vi "PSCHN_Update Variable.vi"(6 "data":cluster{"Tag":string, "Popup Value":variant}, 8 "error in (no error)":errorcluster, 9 "PopUp Para":T5, 10 "Cards":T1[](array[typedef]), 11 "Tree":refnum<vi>) -> (0 "error out":errorcluster, 2 "Cards Out":T1[](array[typedef]))   [LabVIEW 2016]
uses:
  Controls/PSCHN_Card Para.ctl
  Controls/PSCHN_Channel Para.ctl
  <vilib>/Pansino Software/ToolkitLib/Popup Toolkit/Private/Ctrls/PSPOP_Grid.Cell Info.ctl
  <vilib>/Pansino Software/ToolkitLib/Popup Toolkit/Private/Ctrls/PSPOP_Data Type.ctl
panel:
  in  "Cell Info (type only)":T3={"Tag"="", "Row"=0, "Column"=0, "In Symbol?"=FALSE, "In Data?"=FALSE, "Cell String"="", "Ctl Refnum"=refnum, "Prop Type"=enum."Unkown", "Ring Strings"=[], "Ring Values"=[], "New Cell String"=""}
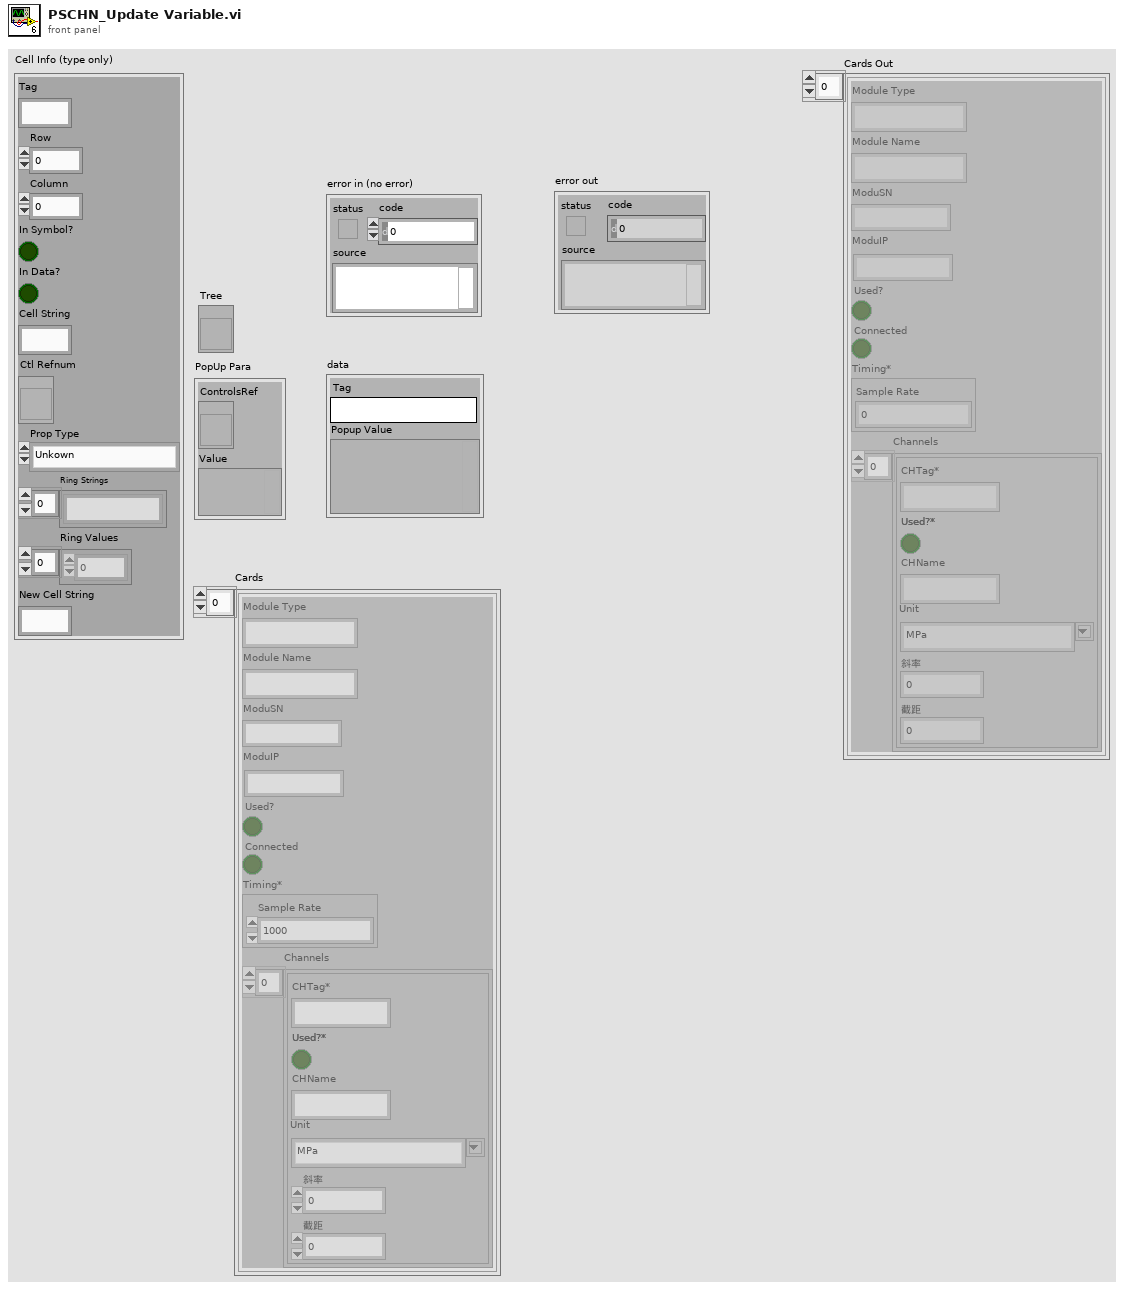
[diagram p1: front panel]
types:
  T1 = typedef "PSCHN_Card Para.ctl" = cluster{"Module Type":string, "Module Name":string, "ModuSN":string, "ModuIP":string, "Used?":bool, "Connected":bool, "Timing*":cluster{"Sample Rate":dbl}, "Channels":T2[]}
  T2 = typedef "PSCHN_Channel Para.ctl" = cluster{"CHTag*":string, "Used?*":bool, "CHName":string, "Unit":string, "斜率":dbl, "截距":dbl}
  T3 = typedef "PSPOP_Grid.Cell Info.ctl" = cluster{"Tag":string, "Row":i32, "Column":i32, "In Symbol?":bool, "In Data?":bool, "Cell String":string, "Ctl Refnum":refnum<vi>, "Prop Type":T4, "Ring Strings":string[], "Ring Values":ext[], "New Cell String":string}
  T4 = typedef "PSPOP_Data Type.ctl" = enum16{"NO POPUP", "Unkown", "String", "Integer", "Float", "Color", "Boolean", "Ring", "Captioned String", "Captioned Integer", "Button Color", "2 Int Cluster", "4 Int Cluster", "6-Dbl Cluster", "Path", "Combox", "Time", "ShotCut String"}
  T5 = cluster{"ControlsRef":refnum<vi>, "Value":variant}
  T6 = typedef "PSCFO_ParaDataType.ctl" = cluster{"ParaTag":string, "ParaName":string, "ParaType":string, "PicName":string, "ParaLevel":string, "DefaultValue":variant, "ParaVisable?":bool, "ParaOperation?":bool, "Operation":cluster{"ParaValue":string, "Operation":cluster{"ChangePara":cluster{"ParaName":string, "ParaData":string}[], "EnablePara":string[]}}[], "Ring Para":T7}
  T7 = typedef "PSLIST_Para Related.ctl" = cluster{"Strings":string[], "Values":ext[], "Use":bool, "Combox":string[], "Browse Options":T8, "Combo Box":cluster{"Allow Undefined Strings":bool}}
  T8 = typedef "LVBrowseOptionsTypeDef.ctl" = cluster{"Prompt":string, "Match Pattern":string, "Mode":enum32{"existing file", "new file", "new or existing file", "existing dir", "new dir", "new or existing dir", "existing file (use LLBs)", "new file (use LLBs)", "new or existing file (use LLBs)", "new or existing file or directory (use LLBs)", "existing dir (use LLBs)", "new dir (use LLBs)", "new or existing dir (use LLBs)", "existing file or dir", "new file or dir", "new or existing file or dir", "existing file or dir (use LLBs)", "new file or dir (use LLBs)"}, "Start Path":path, "Pattern Label":string, "Button Text":string}
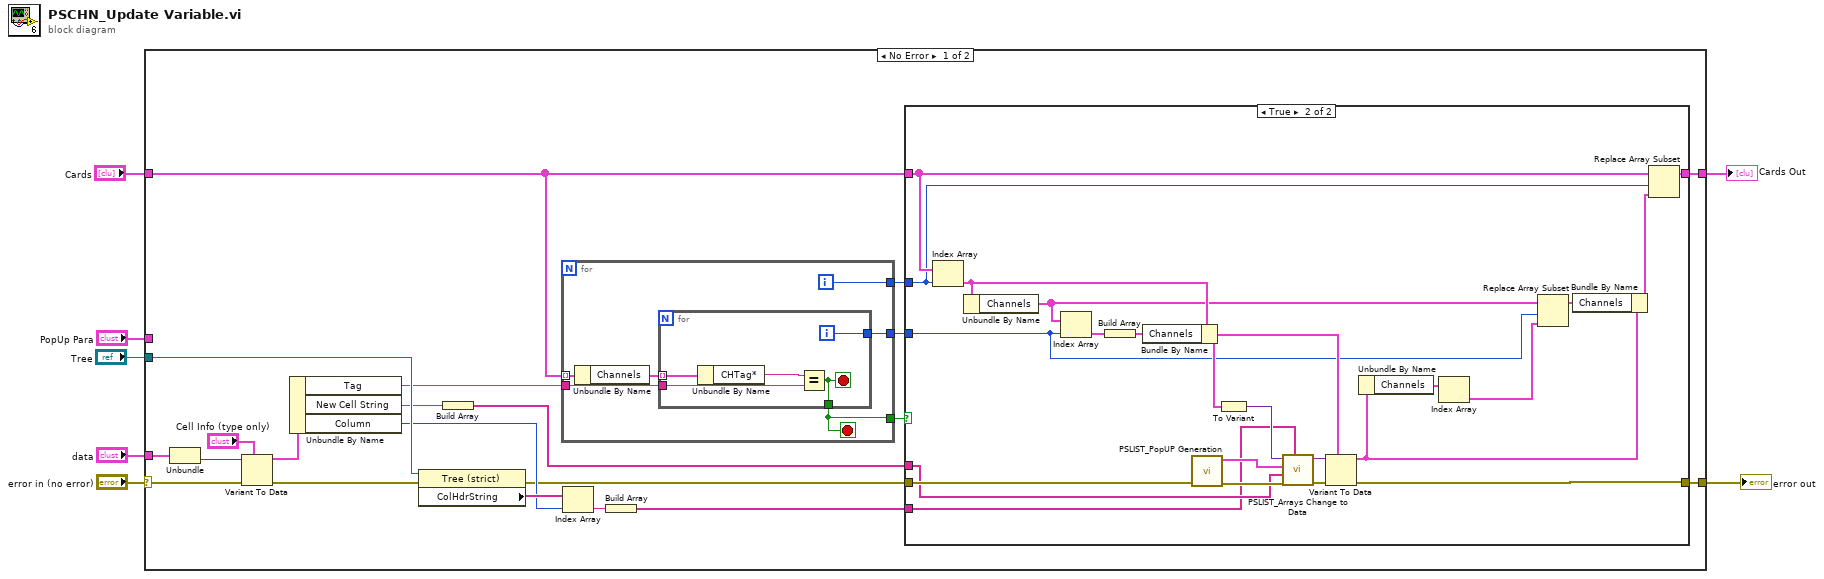
[diagram p0: block diagram]
diagram:
  n1 = case shown="No Error" "error in (no error)" {
    selector: "error in (no error)" -> [w27 w66]
    tunnel: [w12 w66] -> w7
    tunnel: "PopUp Para" -> [_ _]
    tunnel: "Cards" -> [w15 w65]
    tunnel: "data" -> [w28 _]
    tunnel: "Tree" -> [w23 _]
    tunnel: [w14 w65] -> w1
    frame No Error {
      n2 = Unbundle(w28) -> ("Popup Value"=w26:variant)  [unwired: 1 out]
      n3 = Variant To Data(error in=w27, type="Cell Info (type only)", Variant=w26) -> (data=w24:T3, error out=w22:errorcluster)
      n4 = Unbundle By Name(w24) -> ("Tag"=w19:string, "New Cell String"=w18:string, "Column"=w20:i32)
      n5 = property class="Tree (strict)"(reference=w23, error in=w22) -> (error out=w13:errorcluster, "ColHdrString"=w21:string[])  [unwired: 1 out]
      n6 = Build Array(w18) -> (w8:string[])
      n7 = for {
        tunnel: w15 -> [w57] mode=indexing
        tunnel: w19 -> [w58]
        tunnel: [w56] -> w10
        tunnel: [w55] -> w11
        tunnel: [w54] -> w16
        i -> [w55]
        stop <- w54 stop-if-true
        n8 = Unbundle By Name(w57) -> ("Channels"=w59:T2[])
        n9 = for {
          tunnel: w59 -> [w62] mode=indexing
          tunnel: w58 -> [w63]
          tunnel: [w61] -> w54
          tunnel: [w60] -> w56
          i -> [w60]
          stop <- w61 stop-if-true
          n10 = Unbundle By Name(w62) -> ("CHTag*"=w64:string)
          n11 = Equal?(x=w64, y=w63) -> (x = y?=w61:bool)
        }
      }
      n12 = Index Array(array=w21, index=w20) -> (element=w17:string)
      n13 = Build Array(w17) -> (w9:string[])
      n14 = case shown="True" w16 {
        tunnel: w15 -> [w30 w37]
        tunnel: [w30 w34] -> w14
        tunnel: w13 -> [w29 w50]
        tunnel: [w29 w32] -> w12
        tunnel: w11 -> [_ w36]
        tunnel: w10 -> [_ w40]
        tunnel: w9 -> [_ w33]
        tunnel: w8 -> [_ w42]
        frame False {
        }
        frame True {
          n15 = Index Array(array=w37, index=w36) -> (element=w51:T1)
          n16 = Unbundle By Name(w51) -> ("Channels"=w41:T2[])
          n17 = Index Array(array=w41, index=w40) -> (element=w52:T2)
          n18 = Build Array(w52) -> (w53:T2[])
          n19 = Bundle By Name(cluster=w51, "Channels"=w53) -> (w49:T1)
          n20 = call <vilib>:"PSLIST_PopUP Generation.vi"("错误输入（无错误）"=w50) -> ("error out"=w45:errorcluster, "PopUpPara"=w44:T6[])  [unwired: 9 in]
          n21 = To Variant(anything=w49) -> (Variant=w46:variant)
          n22 = call <vilib>:"PSLIST_Arrays Change to Data.vi"("Column Headers"=w33, "Error In"=w45, "Column Strings"=w42, "Parameter"=w44, "VData"=w46) -> ("Error Out"=w47:errorcluster, "Data Out"=w48:variant)  [unwired: 4 in, 1 out]
          n23 = Variant To Data(error in=w47, type=w49, Variant=w48) -> (data=w39:T1, error out=w32:errorcluster)
          n24 = Unbundle By Name(w39) -> ("Channels"=w43:T2[])
          n25 = Index Array(array=w43) -> (element=w31:T2)  [unwired: 1 in]
          n26 = Replace Array Subset(array=w41, new element=w31, index=w40) -> (w38:T2[])
          n27 = Bundle By Name(cluster=w39, "Channels"=w38) -> (w35:T1)
          n28 = Replace Array Subset(array=w37, new element=w35, index=w36) -> (w34:T1[])
        }
      }
    }
    frame Error {
    }
  }
  "error out" <- w7
  "Cards Out" <- w1
